vi "sub_NMEA_linefeed_cut.vi"(11 "GPS raw data buffer":string) -> (1 "GNVTG":string, 2 "GNRMC":string, 3 "GNGGA ($제거 문자열)":string)   [LabVIEW 2020]
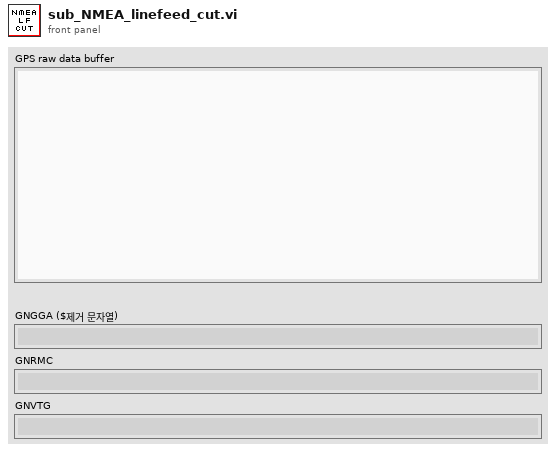
[diagram p1: front panel]
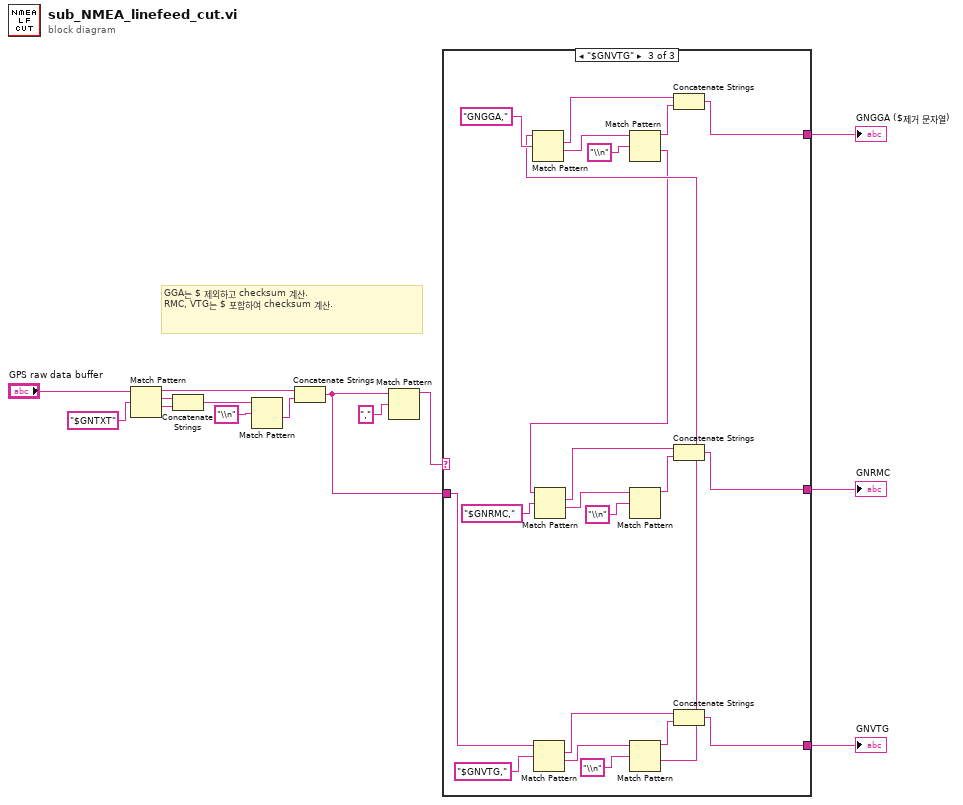
[diagram p0: block diagram]
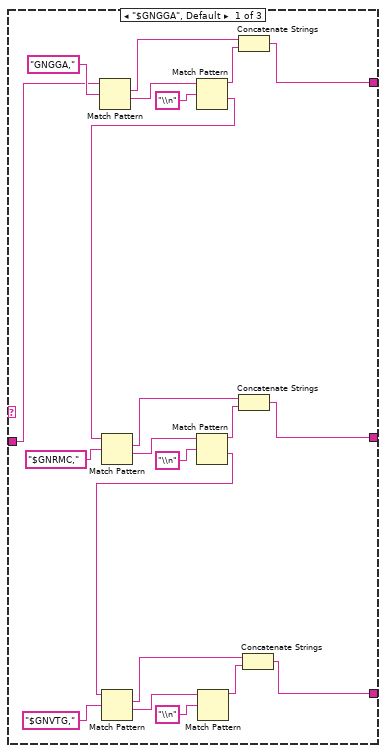
[diagram p2: hidden frame]
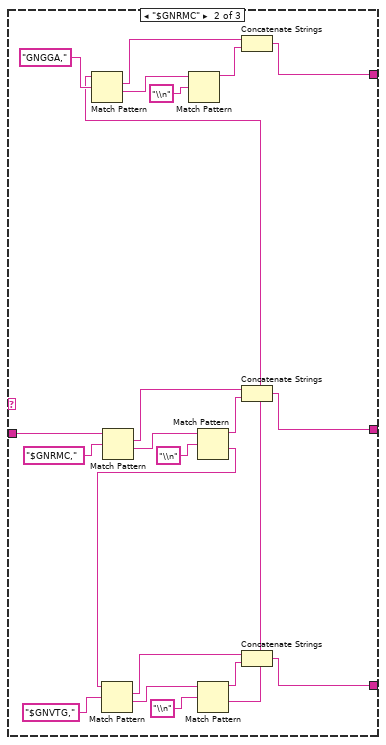
[diagram p3: hidden frame]
diagram:
  # "GGA는 $ 제외하고 checksum 계산.\nRMC, VTG는 $ 포함하여 checksum 계산."
  n1 = Match Pattern(string="GPS raw data buffer", regular expression="$GNTXT" ("정규식")) -> (before substring=w3:string, match substring=w7:string, after substring=w6:string)  [unwired: 1 in, 1 out]
  n2 = Concatenate Strings(w7, w6) -> (w5:string)
  n3 = Match Pattern(string=w5, regular expression="\\n" ("정규식")) -> (after substring=w2:string)  [unwired: 1 in, 3 out]
  n4 = Concatenate Strings(w3, w2) -> (w1:string)
  n5 = Match Pattern(string=w1, regular expression="," ("정규식")) -> (before substring=w11:string)  [unwired: 1 in, 3 out]
  n6 = case shown="\"$GNVTG\"" w11 {
    tunnel: w1 -> [w26 w50 w67]
    tunnel: [w21 w44 w65] -> w12
    tunnel: [w19 w41 w64] -> w13
    tunnel: [w17 w38 w63] -> w14
    frame "$GNGGA", Default {
      n7 = Match Pattern(string=w26, regular expression="GNGGA," ("정규식")) -> (match substring=w23:string, after substring=w25:string)  [unwired: 1 in, 2 out]
      n8 = Match Pattern(string=w25, regular expression="\\n" ("검색 문자열/문자 (-)")) -> (before substring=w22:string, after substring=w28:string)  [unwired: 1 in, 2 out]
      n9 = Match Pattern(string=w28, regular expression="$GNRMC," ("정규식")) -> (match substring=w18:string, after substring=w27:string)  [unwired: 1 in, 2 out]
      n10 = Match Pattern(string=w27, regular expression="\\n" ("검색 문자열/문자 (-)")) -> (before substring=w20:string, after substring=w24:string)  [unwired: 1 in, 2 out]
      n11 = Match Pattern(string=w24, regular expression="$GNVTG," ("정규식")) -> (match substring=w15:string, after substring=w30:string)  [unwired: 1 in, 2 out]
      n12 = Match Pattern(string=w30, regular expression="\\n" ("검색 문자열/문자 (-)")) -> (before substring=w16:string)  [unwired: 1 in, 3 out]
      n13 = Concatenate Strings(w23, w22) -> (w21:string)
      n14 = Concatenate Strings(w18, w20) -> (w19:string)
      n15 = Concatenate Strings(w15, w16) -> (w17:string)
    }
    frame "$GNRMC" {
      n16 = Match Pattern(string=w50, regular expression="$GNRMC," ("정규식")) -> (match substring=w39:string, after substring=w51:string)  [unwired: 1 in, 2 out]
      n17 = Match Pattern(string=w51, regular expression="\\n" ("검색 문자열/문자 (-)")) -> (before substring=w40:string, after substring=w46:string)  [unwired: 1 in, 2 out]
      n18 = Match Pattern(string=w46, regular expression="$GNVTG," ("정규식")) -> (match substring=w36:string, after substring=w53:string)  [unwired: 1 in, 2 out]
      n19 = Match Pattern(string=w53, regular expression="\\n" ("검색 문자열/문자 (-)")) -> (before substring=w37:string, after substring=w45:string)  [unwired: 1 in, 2 out]
      n20 = Match Pattern(string=w45, regular expression="GNGGA," ("정규식")) -> (match substring=w42:string, after substring=w47:string)  [unwired: 1 in, 2 out]
      n21 = Match Pattern(string=w47, regular expression="\\n" ("검색 문자열/문자 (-)")) -> (before substring=w43:string)  [unwired: 1 in, 3 out]
      n22 = Concatenate Strings(w42, w43) -> (w44:string)
      n23 = Concatenate Strings(w39, w40) -> (w41:string)
      n24 = Concatenate Strings(w36, w37) -> (w38:string)
    }
    frame "$GNVTG" {
      n25 = Match Pattern(string=w67, regular expression="$GNVTG," ("정규식")) -> (match substring=w57:string, after substring=w74:string)  [unwired: 1 in, 2 out]
      n26 = Match Pattern(string=w74, regular expression="\\n" ("검색 문자열/문자 (-)")) -> (before substring=w58:string, after substring=w68:string)  [unwired: 1 in, 2 out]
      n27 = Match Pattern(string=w68, regular expression="GNGGA," ("정규식")) -> (match substring=w61:string, after substring=w69:string)  [unwired: 1 in, 2 out]
      n28 = Match Pattern(string=w69, regular expression="\\n" ("검색 문자열/문자 (-)")) -> (before substring=w62:string, after substring=w66:string)  [unwired: 1 in, 2 out]
      n29 = Match Pattern(string=w66, regular expression="$GNRMC," ("정규식")) -> (match substring=w59:string, after substring=w72:string)  [unwired: 1 in, 2 out]
      n30 = Match Pattern(string=w72, regular expression="\\n" ("검색 문자열/문자 (-)")) -> (before substring=w60:string)  [unwired: 1 in, 3 out]
      n31 = Concatenate Strings(w61, w62) -> (w65:string)
      n32 = Concatenate Strings(w59, w60) -> (w64:string)
      n33 = Concatenate Strings(w57, w58) -> (w63:string)
    }
  }
  "GNVTG" <- w14
  "GNRMC" <- w13
  "GNGGA ($제거 문자열)" <- w12
